vi "[RE Python] Day 3.vi"() -> ()   [LabVIEW 2019]
panel:
  out "Claim Without Overlap":i32
  out "Fabric":i32[][](array[numeric])
  out "Error Out":errorcluster
  out "Sq in of Overlapping Claims":i32
  out "Elf Claims":string[][](array[string])
  in  "Error In":errorcluster
  in  "Relative Path to Input File":string="Day 3\\Day 3 Raw Input.txt"
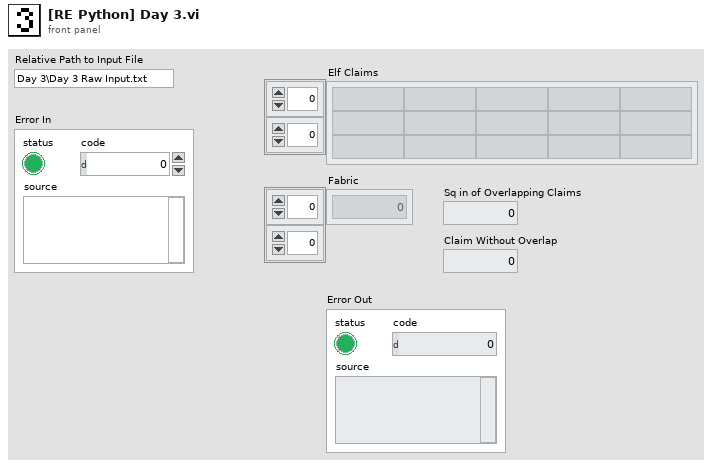
[diagram p1: front panel]
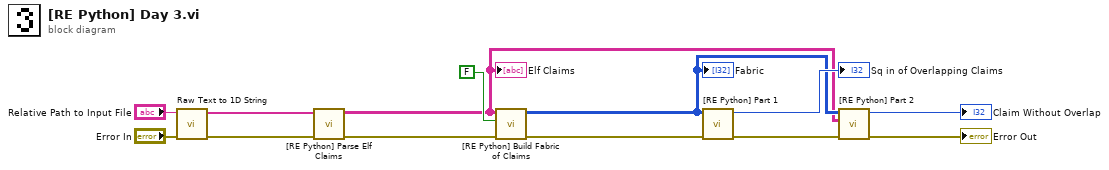
[diagram p0: block diagram]
diagram:
  n1 = call "Raw Text to 1D String.vi"("Error In"="Error In", "Relative Path to Input File"="Relative Path to Input File") -> ("Error Out"=w10:errorcluster, "1D String Array"=w11:string[])  [unwired: 8 in]
  n2 = call "[RE Python] Parse Elf Claims.vi"("error in (no error)"=w10, "1D String Array"=w11) -> ("Error Out"=w9:errorcluster, "Elf Claims"=w4:string[][])  [unwired: 8 in]
  "Elf Claims" <- w4
  n3 = call "[RE Python] Build Fabric of Claims.vi"("Error In"=w9, "Debugging"=FALSE, "Split String"=w4) -> ("Error Out"=w7:errorcluster, "Fabric"=w5:i32[][])  [unwired: 7 in]
  "Fabric" <- w5
  n4 = call "[RE Python] Part 1.vi"("Error In"=w7, "Fabric"=w5) -> ("Error Out"=w2:errorcluster, "Sq in of Overlapping Claims"=→"Sq in of Overlapping Claims":i32)  [unwired: 8 in]
  n5 = call "[RE Python] Part 2.vi"("Error In"=w2, "Elf Claims"=w4, "Fabric"=w5) -> ("Error Out"=→"Error Out":errorcluster, "Claim Without Overlap"=→"Claim Without Overlap":i32)  [unwired: 7 in]
